vi "בדיקת זמן ניתוק הממסר 7.vi"(7 "resultUserPrompt":bool, 8 "error":errorcluster, 11 "Path for Log":path) -> (0 "error out":errorcluster, 1 "בטוח כן/לא":bool, 2 "בדיקת זמן ניתוק הממסר":dbl)   [LabVIEW 2014]
uses:
  <instrlib>/niDMM/nidmm.llb/niDMM Function.ctl
  <instrlib>/niDMM/nidmm.llb/niDMM Resolution in Digits.ctl
  <vilib>/DAQmx/create/channels.llb/DAQmx Create Channel (DO-Digital Output).vi
  <vilib>/DAQmx/write.llb/DAQmx Write (Digital Bool 1Line 1Point).vi
  <instrlib>/niDMM/nidmm.llb/niDMM Configure Measurement Digits.vi
panel:
  # "Right-Click to\nexplain error"
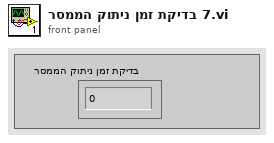
[diagram p1: front panel]
types:
  T1 = enum32{"Invalid", "Standard", "Closed", "Hidden", "Minimized", "Maximized"}
  T2 = typedef "niDMM Function.ctl" = enum16{"DC Volts", "AC Volts", "DC Current", "AC Current", "2-wire Resistance", "4-wire Resistance", "Diode", "Frequency", "Period", "AC Volts DC Coupled", "Capacitance", "Inductance", "Temperature"}
  T3 = typedef "niDMM Resolution in Digits.ctl" = dbl
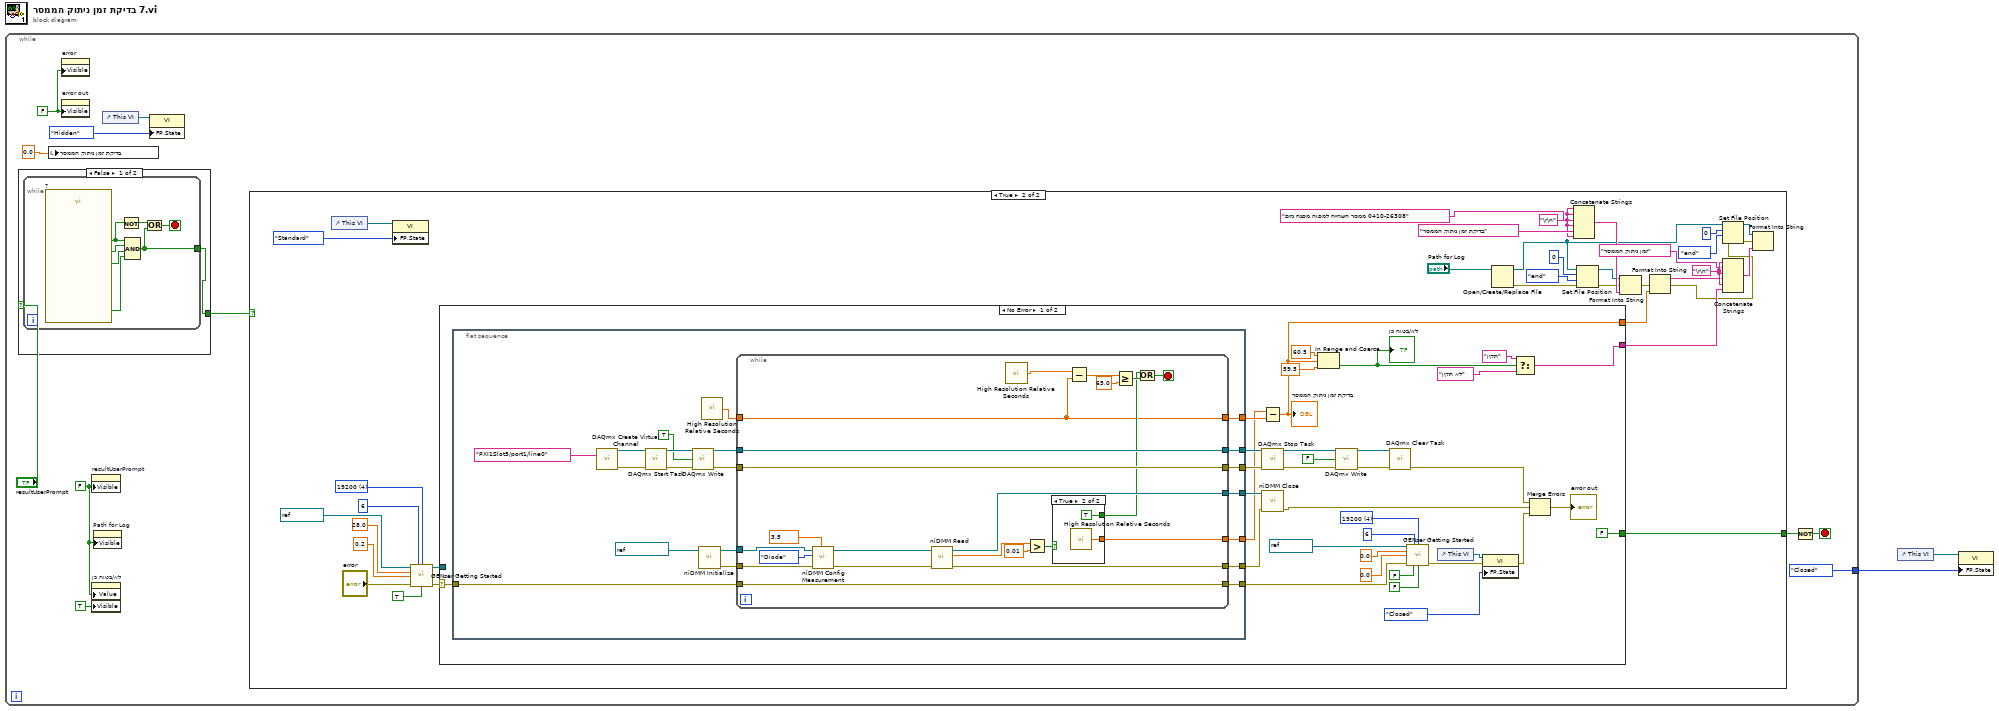
[diagram p0: block diagram]
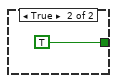
[diagram p2: hidden frame]
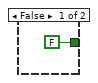
[diagram p3: hidden frame]
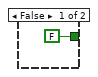
[diagram p4: hidden frame]
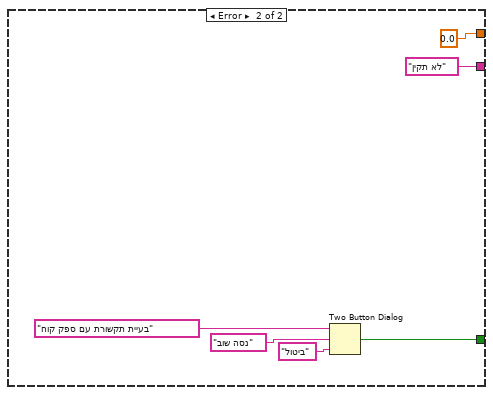
[diagram p5: hidden frame]
diagram:
  n1 = while {
    tunnel: [T1."Closed" ("Front Panel Window:State")] -> w1
    stop <- w12 stop-if-true
    w5 = FALSE ("Visible")
    w10 = FALSE ("Visible")
    n2 = case shown="False" "resultUserPrompt" {
      tunnel: [w14 TRUE] -> w13
      frame False {
        n3 = while {
          tunnel: [w16] -> w14
          stop <- w18 stop-if-true
          n4 = call "?"() -> ("הדקי הרב מודד"=w19:bool, "(מגע שלילי (מעטפת"=w20:bool, "C מגע חיובי"=w21:bool, "OK"=w15:bool)  [unwired: 15 in, 1 out]
          n5 = Not(x=w15) -> (.not. x?=w17:bool)
          n6 = Compound Arithmetic op=AND(w15, w21, w20, w19) -> (w16:bool)
          n7 = Or(x=w17, y=w16) -> (x .or. y?=w18:bool)
        }
      }
      frame True {
      }
    }
    n8 = local write "בדיקת זמן ניתוק הממסר"(0.0 ("זמן ניתוק הממסר")) -> ()
    n9 = property on="error" class="Clust (strict)"("Visible"=w10) -> ()  [unwired: 2 in, 2 out]
    n10 = property on="error out" class="Clust (strict)"("Visible"=w10) -> ()  [unwired: 2 in, 2 out]
    n11 = property on="resultUserPrompt" class="Bool (strict)"("Visible"=w5) -> ()  [unwired: 2 in, 2 out]
    n12 = property on="בטוח כן/לא" class="Bool (strict)"("Value"=w5, "Visible"=TRUE) -> ()  [unwired: 2 in, 2 out]
    n13 = property on="Path for Log" class="Path"("Visible"=w5) -> ()  [unwired: 2 in, 2 out]
    n14 = control-ref of="This VI"() -> (w9:refnum<vi>)
    n15 = property class="VI"(reference=w9, "FP.State"=T1."Hidden" ("Front Panel Window:State")) -> ()  [unwired: 1 in, 2 out]
    n16 = case shown="True" w13 {
      tunnel: [FALSE ("T button?") w51] -> w11
      frame False {
      }
      frame True {
        w33 = "\r\n"
        w41 = "\r\n"
        w55 = u16 4 items=["1200", "2400", "4800", "9600", "19200"] ("BAUD")
        n17 = control-ref of="This VI"() -> (w50:refnum<vi>)
        n18 = property class="VI"(reference=w50, "FP.State"=T1."Standard" ("Front Panel Window:State")) -> ()  [unwired: 1 in, 2 out]
        n19 = call "GENser Getting Started.vi"("VISA"=refnum<visa-resource-name> "COM6", "GEN Addr"=i16 6, "BAUD"=w55, "Voltage Limit"=28.0, "Current Limit"=0.2, "error"="error", "Output On (T)"=TRUE) -> ("VISA out"=w56:refnum<visa-resource-name>, "error out"=w47:errorcluster)  [unwired: 5 in, 2 out]
        n20 = case shown="No Error" w47 {
          selector: w47 -> [w85 _]
          tunnel: w56 -> [_ _]
          tunnel: [FALSE ("T button?") w141] -> w51
          tunnel: [w63 0.0] -> w27
          tunnel: [w59 "לא תקין"] -> w26
          frame No Error {
            w80 = u16 4 items=["1200", "2400", "4800", "9600", "19200"] ("BAUD")
            n21 = flat-sequence {
              tunnel: [w107] -> w64
              tunnel: [w106] -> w65
              tunnel: [w105] -> w72
              tunnel: [w104] -> w73
              tunnel: [w103] -> w69
              tunnel: w85 -> [w102]
              tunnel: [w101] -> w84
              tunnel: [w100] -> w70
              frame #0 {
                n22 = call-poly <vilib>:"DAQmx Create Virtual Channel.vi"("lines"=tag "PXI1Slot5/port1/line0") -> ("task out"=w109:refnum<k21>, "error out"=w110:errorcluster)  [unwired: 13 in]
                n23 = call <vilib>:"DAQmx Start Task.vi"("task/channels in"=w109, "error in"=w110) -> ("task out"=w99:refnum<k21>, "error out"=w98:errorcluster)  [unwired: 12 in]
                n24 = call-poly <vilib>:"DAQmx Write.vi"("task/channels in"=w99, "data"=TRUE, "error in"=w98) -> ("task out"=w96:refnum<k21>, "error out"=w97:errorcluster)  [unwired: 10 in, 1 out]
                n25 = call <instrlib>:"niDMM Initialize.vi"("Instrument Descriptor"=refnum<k15> "PXI1Slot9") -> ("error out"=w111:errorcluster, "instrument handle out"=w112:refnum<k15>)  [unwired: 9 in]
                n26 = call <vilib>:"High Resolution Relative Seconds.vi"() -> ("relative seconds"=w94:dbl)
                n27 = while {
                  tunnel: [w115] -> w106
                  tunnel: [w133] -> w107
                  tunnel: [w126] -> w103
                  tunnel: [w118] -> w104
                  tunnel: [w117] -> w105
                  tunnel: [w125] -> w100
                  tunnel: w112 -> [w130]
                  tunnel: w111 -> [w129]
                  tunnel: w96 -> [w118]
                  tunnel: w97 -> [w117]
                  tunnel: [w119] -> w101
                  tunnel: w102 -> [w119]
                  tunnel: w94 -> [w115]
                  stop <- w122 stop-if-true
                  w135 = T3 3.5 items=["3 1/2"=3.5, "4 1/2"=4.5, "5 1/2"=5.5, "6 1/2"=6.5, "7 1/2"=7.5] ("Resolution in Digits")
                  n28 = call-poly <instrlib>:"niDMM Config Measurement.vi"("Resolution in Digits"=w135, "error in (no error)"=w129, "Function"=niDMM_Function."Diode", "instrument handle"=w130) -> ("error out"=w127:errorcluster, "instrument handle out"=w128:refnum<k15>)  [unwired: 6 in]
                  n29 = call <instrlib>:"niDMM Read.vi"("error in (no error)"=w127, "instrument handle"=w128) -> ("error out"=w125:errorcluster, "Measurement"=w132:dbl, "instrument handle out"=w126:refnum<k15>)  [unwired: 7 in]
                  n30 = call <vilib>:"High Resolution Relative Seconds.vi"() -> ("relative seconds"=w114:dbl)
                  n31 = Greater?(x=w132, y=0.01) -> (0:w120:bool)
                  n32 = case shown="True" w120 {
                    tunnel: [_ w138] -> w133
                    tunnel: [FALSE TRUE] -> w116
                    frame False {
                    }
                    frame True {
                      n33 = call <vilib>:"High Resolution Relative Seconds.vi"() -> ("relative seconds"=w138:dbl)
                    }
                  }
                  n34 = Subtract(x=w114, y=w115) -> (x-y=w124:dbl)
                  n35 = Greater Or Equal?(x=w124, y=65.0) -> (x >= y?=w121:bool)
                  n36 = Or(x=w116, y=w121) -> (x .or. y?=w122:bool)
                }
              }
            }
            n37 = Subtract(x=w64, y=w65) -> (x-y=w63:dbl)
            "בדיקת זמן ניתוק הממסר" <- w63
            n38 = call <vilib>:"DAQmx Stop Task.vi"("task/channels in"=w73, "error in"=w72) -> ("task out"=w78:refnum<k21>, "error out"=w77:errorcluster)  [unwired: 12 in]
            n39 = call <instrlib>:"niDMM Close.vi"("error in (no error)"=w70, "instrument handle"=w69) -> ("error out"=w68:errorcluster)  [unwired: 9 in]
            n40 = In Range and Coerce(upper limit=60.5, x=w63, lower limit=59.5) -> (In Range?=w60:bool)  [unwired: 1 out]
            "בטוח כן/לא" <- w60
            n41 = call-poly <vilib>:"DAQmx Write.vi"("task/channels in"=w78, "data"=FALSE, "error in"=w77) -> ("task out"=w75:refnum<k21>, "error out"=w76:errorcluster)  [unwired: 10 in, 1 out]
            n42 = call <vilib>:"DAQmx Clear Task.vi"("task in"=w75, "error in"=w76) -> ("error out"=w71:errorcluster)  [unwired: 13 in]
            n43 = call "GENser Getting Started.vi"("VISA"=refnum<visa-resource-name> "COM6", "GEN Addr"=i16 6, "BAUD"=w80, "Voltage Limit"=0.0, "Current Limit"=0.0, "error"=w84, "Reset (T)"=FALSE ("Output On (T)"), "Output On (T)"=FALSE) -> ("error out"=w86:errorcluster)  [unwired: 4 in, 3 out]
            n44 = control-ref of="This VI"() -> (w88:refnum<vi>)
            n45 = property class="VI"(reference=w88, error in=w86, "FP.State"=T1."Closed" ("Front Panel Window:State")) -> (error out=w82:errorcluster)  [unwired: 1 out]
            n46 = Select(t="תקין", s=w60, f="לא תקין") -> (s? t:f=w59:string)
            n47 = Merge Errors(w71, w68, w82) -> (→"error out":errorcluster)
          }
          frame Error {
            n48 = Two Button Dialog(message="בעיית תקשורת עם ספק קוח", 1:"ביטול" ("F button name (\"Cancel\")"), 2:"נסה שוב" ("T button name (\"OK\")")) -> (T button?=w141:bool)
          }
        }
        n49 = Open/Create/Replace File(file path (use dialog)="Path for Log") -> (refnum out=w28:refnum<file>, error out=w29:errorcluster)  [unwired: 5 in, 1 out]
        n50 = Concatenate Strings(w41, w41, "ממסר השהייה למפוח מפנה גזים 0410-26308", w41, "בדיקת זמן ניתוק הממסר", w41) -> (w44:string)
        n51 = Set File Position(offset (in bytes) (0)=i64 0, refnum=w28, from (0:start)=enum16{"start", "end", "current"}."end", error in=w29) -> (refnum out=w42:refnum<file>, error out=w40:errorcluster)
        n52 = Format Into String(initial string=w42, error in=w40, w44) -> (error out=w39:errorcluster)  [unwired: 1 in, 1 out]
        n53 = Format Into String(error in=w39, w27) -> (resulting string=w31:string, error out=w25:errorcluster)  [unwired: 2 in]
        n54 = Set File Position(offset (in bytes) (0)=i64 0, refnum=w28, from (0:start)=enum16{"start", "end", "current"}."end", error in=w25) -> (refnum out=w36:refnum<file>, error out=w37:errorcluster)
        n55 = Concatenate Strings(w33, "זמן ניתוק הממסר", w33, w31, w33, w26) -> (w38:string)
        n56 = Format Into String(initial string=w36, error in=w37, w38) -> ()  [unwired: 1 in, 2 out]
      }
    }
    n57 = Not(x=w11) -> (.not. x?=w12:bool)
  }
  n58 = control-ref of="This VI"() -> (w2:refnum<vi>)
  n59 = property class="VI"(reference=w2, "FP.State"=w1) -> ()  [unwired: 1 in, 2 out]
